vi "Pre Launch Init.vi"(11 "Nested in":refnum<class "ACQ Generador.lvclass">) -> (0 "error out":errorcluster, 3 "Nested out":refnum<class "ACQ Generador.lvclass">)   [LabVIEW 2020, in "ACQ Generador.lvlib" / "ACQ Generador.lvclass"]
doc: "(<B>Filename</B>: Actor Framework.lvlib:Actor.lvclass:Pre Launch Init.vi)\n\nDefines behavior that occurs after the Launch Nested Actor method is invoked but before the actor's Actor Core method begins running.\n\nBy default, this method does nothing. A descendant class may override it to define behavior."
uses:
  ACQ Generador.lvclass
  ACQ Generador.lvclass/ACQ Generador.ctl
  <vilib>/ActorFramework/Actor/Actor.lvclass
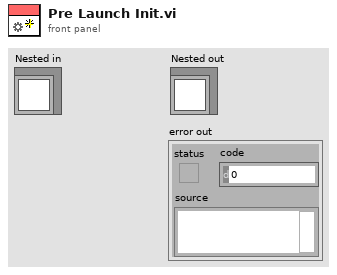
[diagram p1: front panel]
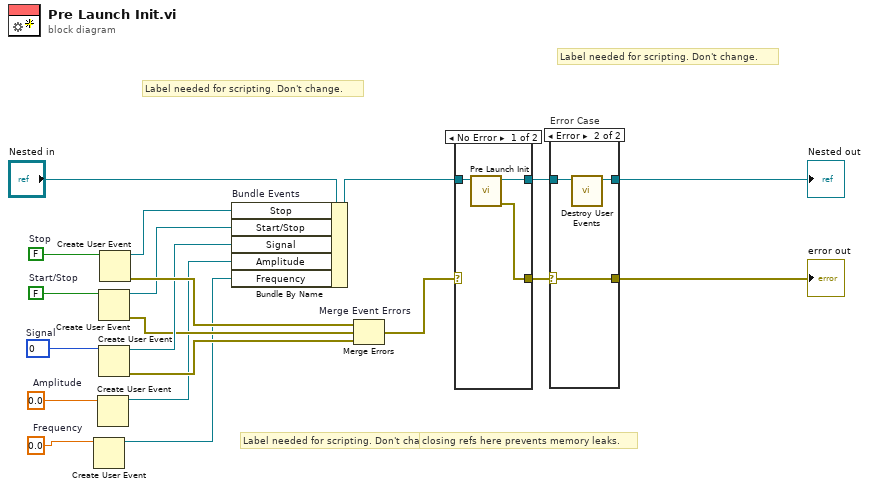
[diagram p0: block diagram]
diagram:
  w1 = 0.0  # Frequency
  w3 = 0.0  # Amplitude
  w7 = u16 0 items=[""]  # Signal
  w8 = FALSE  # Start/Stop
  w19 = FALSE  # Stop
  # "Label needed for scripting. Don't change."
  # "Label needed for scripting. Don't change."
  # "Label needed for scripting. Don't change."
  # "closing refs here prevents memory leaks."
  n1 = Create User Event(user event datatype=w1) -> (user event=w2:refnum<user-event>)  [unwired: 1 in, 1 out]
  n2 = Create User Event(user event datatype=w3) -> (user event=w4:refnum<user-event>)  [unwired: 1 in, 1 out]
  n3 = Create User Event(user event datatype=w8) -> (user event=w10:refnum<user-event>, error out=w6:errorcluster)  [unwired: 1 in]
  n4 = Create User Event(user event datatype=w7) -> (user event=w9:refnum<user-event>, error out=w5:errorcluster)  [unwired: 1 in]
  n5 = Create User Event(user event datatype=w19) -> (user event=w16:refnum<user-event>, error out=w18:errorcluster)  [unwired: 1 in]
  n6 = Bundle By Name "Bundle Events"(cluster="Nested in", "Stop"=w16, "Start/Stop"=w10, "Signal"=w9, "Amplitude"=w4, "Frequency"=w2) -> (w13:refnum<class "ACQ Generador.lvclass">)
  n7 = Merge Errors "Merge Event Errors"(w18, w6, w5) -> (w12:errorcluster)
  n8 = case shown="No Error" w12 {
    selector: w12 -> [_ w25]
    tunnel: [w23 w24] -> w14
    tunnel: w13 -> [w22 w24]
    tunnel: [w21 w25] -> w11
    frame No Error {
      n9 = call-parent "Pre Launch Init.vi"("Actor in"=w22) -> ("error out"=w21:errorcluster, "Actor out"=w23:refnum<class "ACQ Generador.lvclass">)  [unwired: 9 in]
    }
    frame Error {
    }
  }
  n10 = case "Error Case" shown="Error" w11 {
    selector: w11 -> [w26 w30]
    tunnel: w14 -> [w27 w29]
    tunnel: [w27 w28] -> w17
    tunnel: [w26 w30] -> w15
    frame No Error {
    }
    frame Error {
      n11 = call "Destroy User Events.vi"("UI Template in"=w29) -> ("UI Template out"=w28:refnum<class "ACQ Generador.lvclass">)  [unwired: 10 in]
    }
  }
  "error out" <- w15
  "Nested out" <- w17
